vi "XYZTheta-2Zspeed Go.vi"(8 "error in (no error)":errorcluster, 10 "XYZTheta In":dbl[](array[numeric]), 11 "Motion in":refnum<class "Motion.lvclass">) -> (0 "error out":errorcluster, 2 "XYZTheta Out":dbl[](array[numeric]), 3 "Motion out":refnum<class "Motion.lvclass">)   [LabVIEW 2016, in "Motion.lvclass"]
uses:
  Motion.lvclass
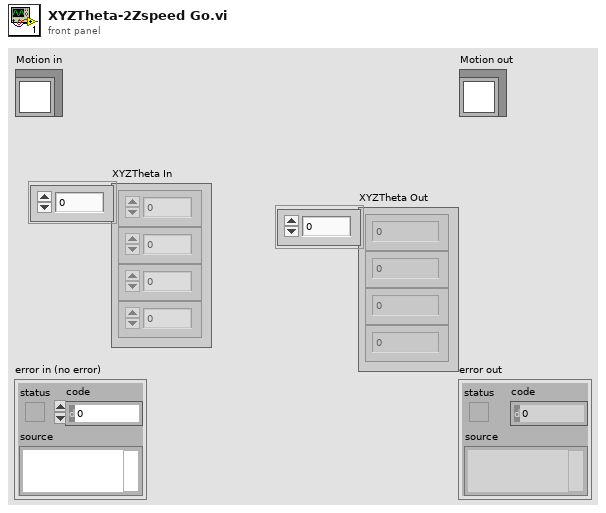
[diagram p1: front panel]
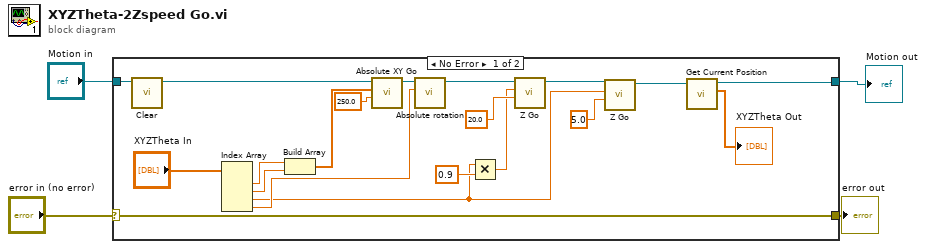
[diagram p0: block diagram]
diagram:
  n1 = case shown="No Error" "error in (no error)" {
    selector: "error in (no error)" -> [w24 w26]
    tunnel: [w24 w26] -> w1
    tunnel: [w6 w25] -> w3
    tunnel: "Motion in" -> [w23 w25]
    frame No Error {
      n2 = call "Clear.vi"("Motion in"=w23) -> ("Motion out"=w21:refnum<class "Motion.lvclass">)  [unwired: 9 in, 1 out]
      n3 = Index Array(array="XYZTheta In") -> (element #1=w14:dbl, element #2=w13:dbl, element #3=w9:dbl, element #4=w22:dbl)  [unwired: 4 in]
      n4 = Build Array(w14, w13) -> (w20:dbl[])
      n5 = call-dynamic "Absolute XY Go.vi"("Speed"=250.0, "XY"=w20, "Motion in"=w21) -> ("Motion out"=w18:refnum<class "Motion.lvclass">)  [unwired: 7 in, 1 out]
      n6 = call-dynamic "Absolute rotation.vi"("Theta"=w22, "Motion in"=w18) -> ("Motion out"=w17:refnum<class "Motion.lvclass">)  [unwired: 8 in, 1 out]
      n7 = Multiply(x=w9, y=0.9) -> (x*y=w8:dbl)
      n8 = call-dynamic "Z Go.vi"("Speed"=20.0, "Position"=w8, "Motion in"=w17) -> ("Motion out"=w12:refnum<class "Motion.lvclass">)  [unwired: 7 in, 1 out]
      n9 = call-dynamic "Z Go.vi"("Speed"=5.0, "Position"=w9, "Motion in"=w12) -> ("Motion out"=w7:refnum<class "Motion.lvclass">)  [unwired: 7 in, 1 out]
      n10 = call-dynamic "Get Current Position.vi"("Motion in"=w7) -> ("XYZTheta Out"=→"XYZTheta Out":dbl[], "Motion out"=w6:refnum<class "Motion.lvclass">)  [unwired: 8 in, 1 out]
    }
    frame Error {
    }
  }
  "error out" <- w1
  "Motion out" <- w3
